vi "NI-XNET Monitor Exit.vi"(8 "Error In":errorcluster, 11 "Process  Data In":T1) -> (0 "Error Out":errorcluster, 3 "Process  Data Out":T1)   [LabVIEW 2017, in "NI-XNET Monitor Engine.lvlib"]
uses:
  NI-XNET Monitor Engine.lvlib
  RTMonitorRefnums.ctl
  <vilib>/NI/NIVS Inline Async API/_Data Access Engine/Data Access Engine/Types/Write.DVR.ctl
  <vilib>/NI/NIVS Inline Async API/_Data Access Engine/Access Type Classes/Write/Write.lvclass
  <vilib>/NI VeriStand/Custom Device Tools/Custom Device Utility Library/Custom Device Utility Library.lvlib
  <vilib>/NI/NIVS Inline Async API/_Data Access Engine/Data Access Engine/Data Access Engine.lvclass
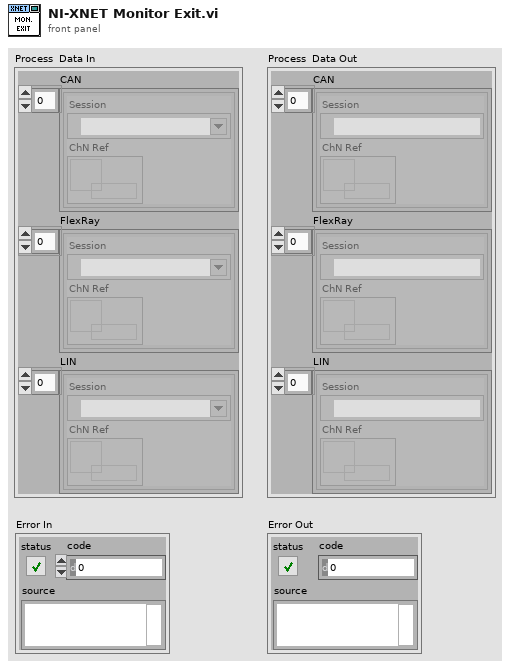
[diagram p1: front panel]
types:
  T1 = typedef "NI-XNET Monitor Engine.lvlib/RTMonitorRefnums.ctl" = cluster{"CAN":cluster{"Session":refnum<k21>, "ChN Ref":T2}[], "FlexRay":cluster{"Session":refnum<k21>, "ChN Ref":T2}[], "LIN":cluster{"Session":refnum<k21>, "ChN Ref":T2}[]}
  T2 = typedef "Data Access Engine.lvlib/Data Access Engine.lvclass/Write.DVR.ctl" = refnum<data-value>
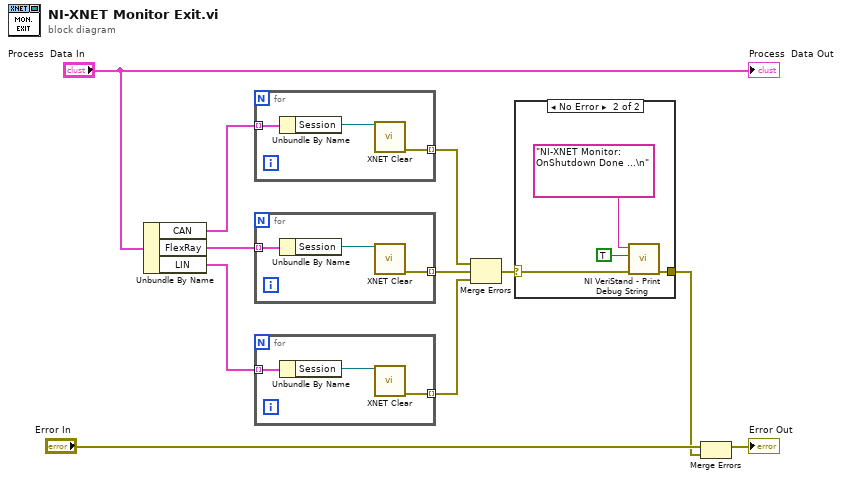
[diagram p0: block diagram]
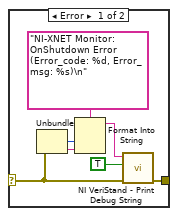
[diagram p2: hidden frame]
diagram:
  n1 = Unbundle By Name("Process  Data In") -> ("CAN"=w8:cluster{"Session":refnum<k21>, "ChN Ref":T2}[], "FlexRay"=w6:cluster{"Session":refnum<k21>, "ChN Ref":T2}[], "LIN"=w5:cluster{"Session":refnum<k21>, "ChN Ref":T2}[])
  n2 = for {
    tunnel: w8 -> [w14] mode=indexing
    tunnel: [w12] -> w7 mode=indexing
    n3 = Unbundle By Name(w14) -> ("Session"=w13:refnum<k21>)
    n4 = call <vilib>:"XNET Clear.vi"("session in"=w13) -> ("error out"=w12:errorcluster)  [unwired: 14 in]
  }
  n5 = for {
    tunnel: w6 -> [w17] mode=indexing
    tunnel: [w15] -> w3 mode=indexing
    n6 = Unbundle By Name(w17) -> ("Session"=w16:refnum<k21>)
    n7 = call <vilib>:"XNET Clear.vi"("session in"=w16) -> ("error out"=w15:errorcluster)  [unwired: 14 in]
  }
  n8 = for {
    tunnel: w5 -> [w20] mode=indexing
    tunnel: [w18] -> w4 mode=indexing
    n9 = Unbundle By Name(w20) -> ("Session"=w19:refnum<k21>)
    n10 = call <vilib>:"XNET Clear.vi"("session in"=w19) -> ("error out"=w18:errorcluster)  [unwired: 14 in]
  }
  n11 = Merge Errors(w7, w3, w4) -> (w2:errorcluster)
  n12 = case shown="No Error" w2 {
    selector: w2 -> [w22 w30]
    tunnel: [w21 w29] -> w1
    frame Error {
      n13 = Unbundle(w22) -> ("code"=w26:i32, "source"=w27:string)  [unwired: 1 out]
      n14 = Format Into String(format string="NI-XNET Monitor: OnShutdown Error (Error_code: %d, Error_msg: %s)\n" ("Message"), w26, w27) -> (resulting string=w25:string)  [unwired: 2 in, 1 out]
      n15 = call <vilib>:"NI VeriStand - Print Debug String.vi"("error in (no error)"=w22, "Add to log file? (T)"=TRUE, "Message"=w25) -> ("error out"=w21:errorcluster)  [unwired: 8 in]
    }
    frame No Error {
      n16 = call <vilib>:"NI VeriStand - Print Debug String.vi"("error in (no error)"=w30, "Add to log file? (T)"=TRUE, "Message"="NI-XNET Monitor: OnShutdown Done ...\n") -> ("error out"=w29:errorcluster)  [unwired: 8 in]
    }
  }
  n17 = Merge Errors("Error In", w1) -> (→"Error Out":errorcluster)
  "Process  Data Out" <- "Process  Data In"
